vi "ReadWFGSettings.vi"(0 "object in":refnum<class "InstrumentBase.lvclass">, 5 "error in (no error)":errorcluster) -> (14 "object out":refnum<class "InstrumentBase.lvclass">, 16 "AmplitudeAndVoltage":T1, 19 "error out":errorcluster)   [LabVIEW 2019, in "InstrumentBase.lvclass"]
uses:
  InstrumentBase.lvclass
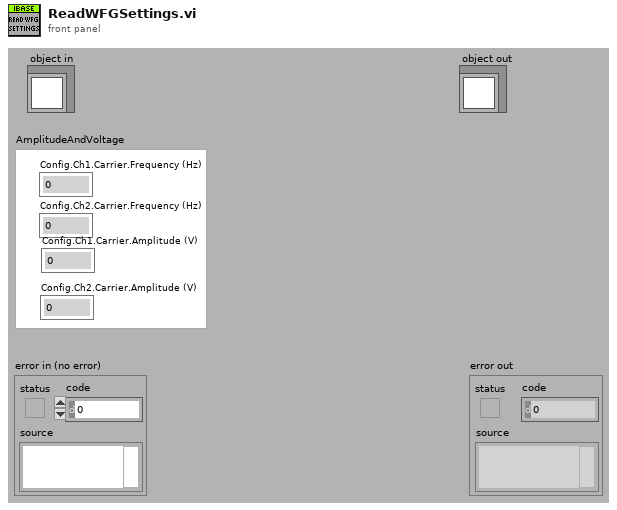
[diagram p1: front panel]
types:
  T1 = cluster{"Config.Ch1.Carrier.Frequency (Hz)":dbl, "Config.Ch2.Carrier.Frequency (Hz)":dbl, "Config.Ch1.Carrier.Amplitude (V)":dbl, "Config.Ch2.Carrier.Amplitude (V)":dbl}
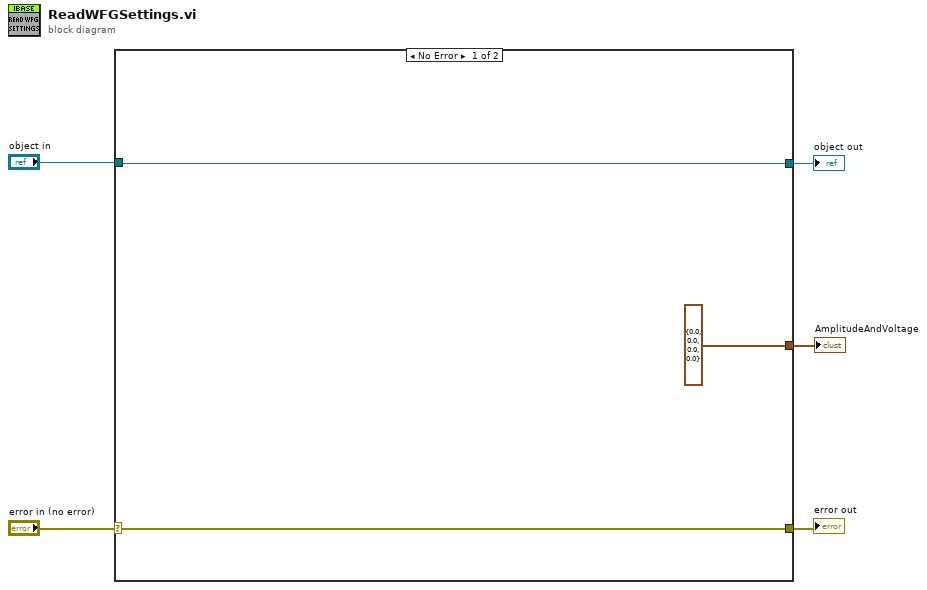
[diagram p0: block diagram]
diagram:
  n1 = case shown="No Error" "error in (no error)" {
    selector: "error in (no error)" -> [w8 w10]
    tunnel: [w8 w10] -> w4
    tunnel: [w7 w9] -> w2
    tunnel: "object in" -> [w7 w9]
    tunnel: [T1 {"Config.Ch1.Carrier.Frequency (Hz)"=0.0, "Config.Ch2.Carrier.Frequency (Hz)"=0.0, "Config.Ch1.Carrier.Amplitude (V)"=0.0, "Config.Ch2.Carrier.Amplitude (V)"=0.0} ("AmplitudeAndVoltage") _] -> w1
    frame No Error {
    }
    frame Error {
    }
  }
  "error out" <- w4
  "object out" <- w2
  "AmplitudeAndVoltage" <- w1
